vi "Bellows Read Position.vi"() -> (0 "Bellows Pos":dbl format="%.9f")   [LabVIEW 2009]
uses:
  MWC Global.vi
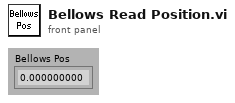
[diagram p1: front panel]
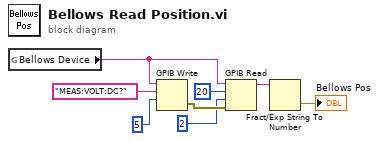
[diagram p0: block diagram]
diagram:
  n1 = global read "MWC Global.vi" "Bellows Device"() -> (w7:string)
  n2 = GPIB Write(0:w7, 1:"MEAS:VOLT:DC?" ("data"), 2:i16 5 ("mode (0)")) -> (6:w6:errorcluster)  [unwired: 2 in, 1 out]
  n3 = GPIB Read(0:w7, 1:20 ("byte count"), 2:i16 2 ("mode (0)"), 3:w6) -> (5:w4:string)  [unwired: 1 in, 2 out]
  n4 = Fract/Exp String To Number(string=w4) -> (number=→"Bellows Pos":dbl)  [unwired: 3 in, 1 out]
